vi "Fetch.vi"(8 "error in (no error)":errorcluster, 11 "VISA resource name":refnum<visa-resource-name>) -> (0 "error out":errorcluster, 2 "Returned Data":string, 3 "VISA resource name out":refnum<visa-resource-name>)   [LabVIEW 2015, in "Agilent 428X Series.lvlib"]
doc: "The Fetch function is sensor-only command which retrieves the measurement data taken by measurement(s) initiate by a trigger, and places the data into the HP 428XA's output buffer."
uses:
  Agilent 428X Series.lvlib
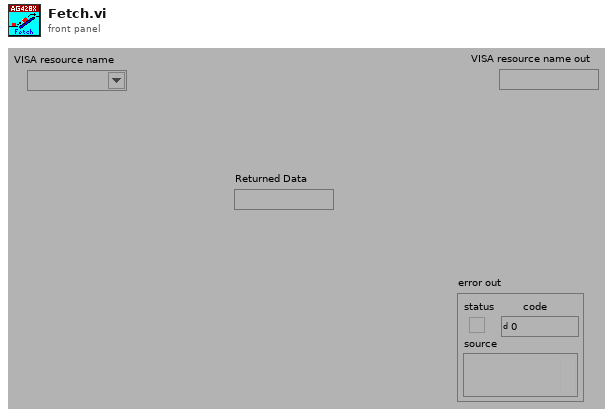
[diagram p1: front panel]
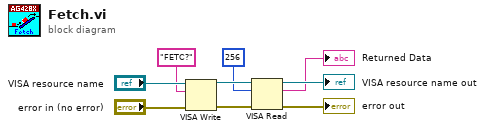
[diagram p0: block diagram]
diagram:
  n1 = VISA Write(VISA resource name="VISA resource name", write buffer="FETC?" ("write buffer (\"\")"), error in (no error)="error in (no error)") -> (VISA resource name out=w8:refnum<visa-resource-name>, error out=w5:errorcluster)  [unwired: 1 out]
  n2 = VISA Read(VISA resource name=w8, byte count=u32 256 ("byte count (0)"), error in (no error)=w5) -> (VISA resource name out=→"VISA resource name out":refnum<visa-resource-name>, read buffer=→"Returned Data":string, error out=→"error out":errorcluster)  [unwired: 1 out]
